vi "S2C_FORNAX_Proc_FormatParameters.vi"(8 "Error In":errorcluster, 9 "CmdName":string, 10 "Type":string, 11 "Cmd":string) -> (0 "Error Out":errorcluster, 1 "RecReturn?":bool, 2 "Returns":string[](array[string]), 3 "Parameters":string[](array[string]))   [LabVIEW 2015]
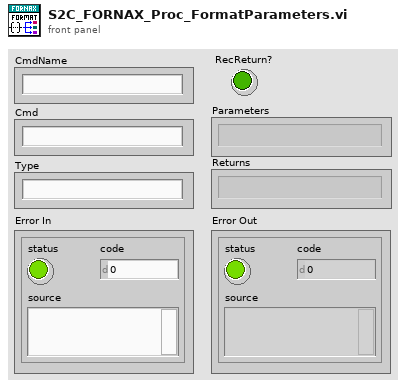
[diagram p1: front panel]
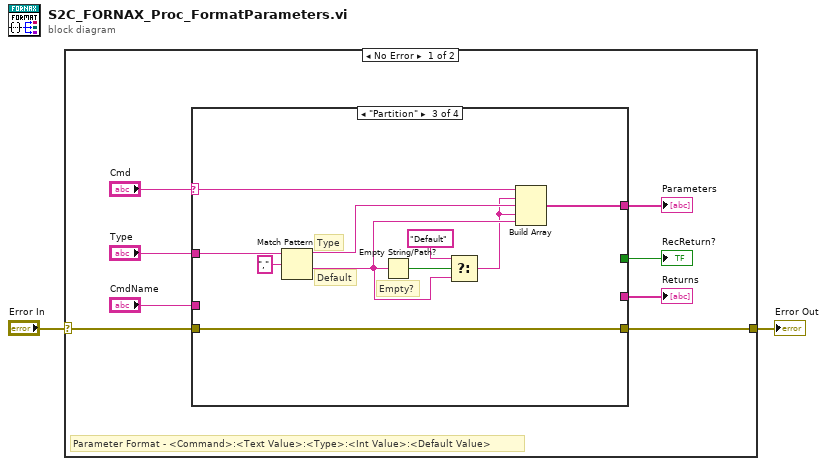
[diagram p0: block diagram]
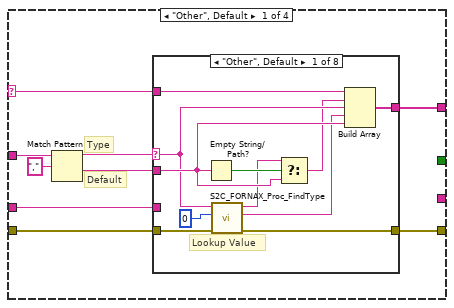
[diagram p2: hidden frame]
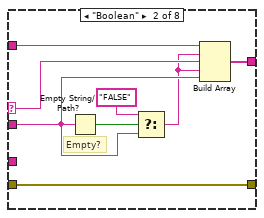
[diagram p3: hidden frame]
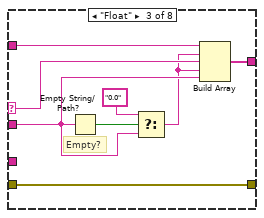
[diagram p4: hidden frame]
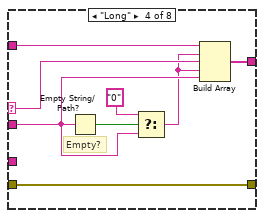
[diagram p5: hidden frame]
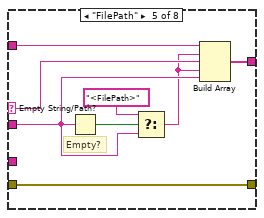
[diagram p6: hidden frame]
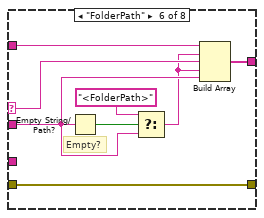
[diagram p7: hidden frame]
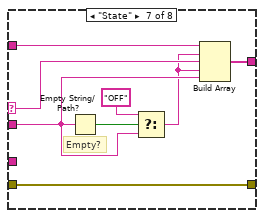
[diagram p8: hidden frame]
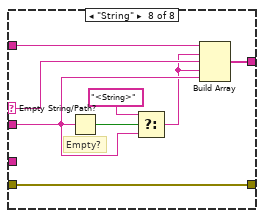
[diagram p9: hidden frame]
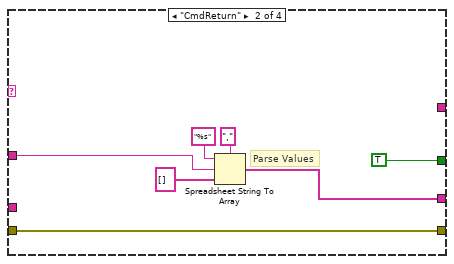
[diagram p10: hidden frame]
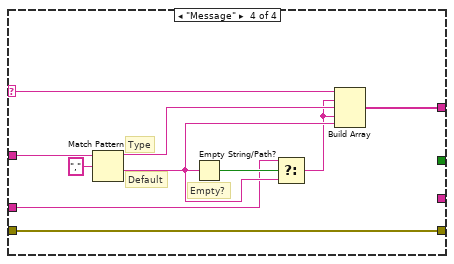
[diagram p11: hidden frame]
diagram:
  n1 = case shown="No Error" "Error In" {
    selector: "Error In" -> [w10 w114]
    tunnel: [w5 w114] -> w1
    frame No Error {
      # "Parameter Format - <Command>:<Text Value>:<Type>:<Int Value>:<Default Value>"
      n2 = case shown="\"Partition\"" "Cmd" {
        selector: "Cmd" -> [w18 _ w103 w113]
        tunnel: w10 -> [w19 w93 w101 w111]
        tunnel: "Type" -> [w15 w92 w99 w109]
        tunnel: "CmdName" -> [w11 _ _ w105]
        tunnel: [w17 _ w102 w112] -> w3
        tunnel: [w16 w93 w101 w111] -> w5
        tunnel: [_ w87 _ _] -> w6
        tunnel: [_ TRUE _ _] -> w4
        frame "Other", Default {
          # "Default"
          # "Type"
          n3 = Match Pattern(string=w15, regular expression=",") -> (before substring=w13:string, after substring=w12:string)  [unwired: 1 in, 2 out]
          n4 = case shown="\"Other\", Default" w13 {
            selector: w13 -> [w23 w33 w41 w49 w57 w65 w73 w81]
            tunnel: w19 -> [w30 w38 w46 w54 w62 w70 w78 w86]
            tunnel: w18 -> [w27 w37 w45 w53 w61 w69 w77 w85]
            tunnel: [w26 w36 w44 w52 w60 w68 w76 w84] -> w17
            tunnel: [w29 w38 w46 w54 w62 w70 w78 w86] -> w16
            tunnel: w12 -> [w24 w32 w40 w48 w56 w64 w72 w80]
            tunnel: w11 -> [_ _ _ _ _ _ _ _]
            frame "Other", Default {
              # "Lookup Value"
              n5 = Empty String/Path?(string/path=w24) -> (empty?=w25:bool)
              n6 = call "S2C_FORNAX_Proc_FindType.vi"("Error In"=w30, "Index"=0, "TypeString"=w23) -> ("Error Out"=w29:errorcluster, "Value_Int"=w22:string, "Value_Text"=w21:string)  [unwired: 4 in, 2 out]
              n7 = Select(t=w21, s=w25, f=w24) -> (s? t:f=w20:string)
              n8 = Build Array(w27, w20, w23, w22, w24) -> (w26:string[])
            }
            frame "Boolean" {
              # "Empty?"
              n9 = Empty String/Path?(string/path=w32) -> (empty?=w35:bool)
              n10 = Select(t="FALSE", s=w35, f=w32) -> (s? t:f=w31:string)
              n11 = Build Array(w37, w31, w33, w31, w32) -> (w36:string[])
            }
            frame "Float" {
              # "Empty?"
              n12 = Empty String/Path?(string/path=w40) -> (empty?=w43:bool)
              n13 = Select(t="0.0", s=w43, f=w40) -> (s? t:f=w39:string)
              n14 = Build Array(w45, w39, w41, w39, w40) -> (w44:string[])
            }
            frame "Long" {
              # "Empty?"
              n15 = Empty String/Path?(string/path=w48) -> (empty?=w51:bool)
              n16 = Select(t="0", s=w51, f=w48) -> (s? t:f=w47:string)
              n17 = Build Array(w53, w47, w49, w47, w48) -> (w52:string[])
            }
            frame "FilePath" {
              # "Empty?"
              n18 = Empty String/Path?(string/path=w56) -> (empty?=w59:bool)
              n19 = Select(t="<FilePath>", s=w59, f=w56) -> (s? t:f=w55:string)
              n20 = Build Array(w61, w55, w57, w55, w56) -> (w60:string[])
            }
            frame "FolderPath" {
              # "Empty?"
              n21 = Empty String/Path?(string/path=w64) -> (empty?=w67:bool)
              n22 = Select(t="<FolderPath>", s=w67, f=w64) -> (s? t:f=w63:string)
              n23 = Build Array(w69, w63, w65, w63, w64) -> (w68:string[])
            }
            frame "State" {
              # "Empty?"
              n24 = Empty String/Path?(string/path=w72) -> (empty?=w75:bool)
              n25 = Select(t="OFF", s=w75, f=w72) -> (s? t:f=w71:string)
              n26 = Build Array(w77, w71, w73, w71, w72) -> (w76:string[])
            }
            frame "String" {
              # "Empty?"
              n27 = Empty String/Path?(string/path=w80) -> (empty?=w83:bool)
              n28 = Select(t="<String>", s=w83, f=w80) -> (s? t:f=w79:string)
              n29 = Build Array(w85, w79, w81, w79, w80) -> (w84:string[])
            }
          }
        }
        frame "CmdReturn" {
          # "Parse Values"
          n30 = Spreadsheet String To Array(delimiter (Tab)=",", format string="%s", spreadsheet string=w92, array type (2D Dbl)=string[] []) -> (array=w87:string[])
        }
        frame "Partition" {
          # "Empty?"
          # "Default"
          # "Type"
          n31 = Match Pattern(string=w99, regular expression=",") -> (before substring=w98:string, after substring=w96:string)  [unwired: 1 in, 2 out]
          n32 = Empty String/Path?(string/path=w96) -> (empty?=w97:bool)
          n33 = Select(t="Default", s=w97, f=w96) -> (s? t:f=w95:string)
          n34 = Build Array(w103, w95, w98, w95, w96) -> (w102:string[])
        }
        frame "Message" {
          # "Empty?"
          # "Default"
          # "Type"
          n35 = Match Pattern(string=w109, regular expression=",") -> (before substring=w108:string, after substring=w106:string)  [unwired: 1 in, 2 out]
          n36 = Empty String/Path?(string/path=w106) -> (empty?=w107:bool)
          n37 = Select(t=w105, s=w107, f=w106) -> (s? t:f=w104:string)
          n38 = Build Array(w113, w104, w108, w104, w106) -> (w112:string[])
        }
      }
      "Parameters" <- w3
      "Returns" <- w6
      "RecReturn?" <- w4
    }
    frame Error {
    }
  }
  "Error Out" <- w1
